vi "subDAQ_SetFilterSet.vi"(6 "Ti-E cluster":T3, 7 "Filterset cluster":T1={"filter set (row)"=18, "Light control ref"=refnum, "Confocal Refnum"=refnum, "DAQ ports"={"Lasers DO lines"=["Dev2/port0/line0", "Dev2/port0/line1", "Dev2/port0/line2", "Dev2/port0/line3", "Dev2/port0/line4", "Dev2/port0/line5"], "Lasers AO lines"=["Dev2/ao0", "Dev2/ao1", "Dev2/ao2", "Dev2/ao3", "Dev2/ao4", "Dev2/ao5"], "Patch AO line"="Dev1/ao1", "Patch AI lines 1"={"Patch scaled output"="Dev1/ai13", "Patch 10 V_m "="Dev1/ai8"}, "Camera timing DI"="Dev1/port0/line23", "Dev1 timing DO "="Dev1/port0/line18", "Dev1 trigger source"="/Dev1/PFI0", "Dev2 trigger source"="/Dev2/PFI0", "LED line"="Dev1/port0/line8", "Global Shutter line"="Dev1/port0/line9", "Patch AI lines 2"={"Cell capacitance"="Dev1/ai9", "Mode"="Dev1/ai10", "Frequency"="Dev1/ai11", "Gain"="Dev1/ai12"}}, "Confocal VISA Setting"="COM1"}, 8 "error in":errorcluster) -> (0 "error out":errorcluster)   [LabVIEW 2015]
uses:
  <vilib>/Analysis/Matrix/Datatypes/RealMatrix.ctl
  <vilib>/Analysis/Matrix/NI_Matrix.lvlib
panel:
  out "Light control":T2={"Filter Set"=17, "Lasers DO"=[TRUE, FALSE, FALSE, FALSE, FALSE, FALSE], "Lasers AO (V)"=[0.3, 0.3, 0.3, 0.3, 0.3, 0.3], "LED"=FALSE, "Global"=TRUE} {"Lasers AO (V)" min=0.0 max=5.0 step=0.01 scale=0.0..5.0 scale format="%#1.2f"; "Filter Set" items=["R-QuasAr", "R-Cy5", "R-mCherry", "R-mOrange", "R-GFP", "R-CFP/DAPI", "R-BFP", "R-LED", "SDC-Cy5", "SDC-mCherry", "SDC-mO2", "SDC-GFP", "SDC-CFP/DAPI", "SDC-BFP", "SDC-LED"]}
  in  "Filter Set Table":T4=[[0.0, 5.0, 2.0, 6.0, 6.0, 1.0, 0.0], [1.0, 0.0, 2.0, 6.0, 6.0, 1.0, 0.0], [2.0, 1.0, 2.0, 2.0, 6.0, 1.0, 0.0], [3.0, 2.0, 1.0, 3.0, 6.0, 1.0, 0.0], [4.0, 3.0, 2.0, 1.0, 6.0, 1.0, 0.0], [5.0, 4.0, 2.0, 5.0, 6.0, 1.0, 0.0], [6.0, 4.0, 2.0, 5.0, 6.0, 1.0, 0.0], [7.0, -1.0, 6.0, 4.0, 6.0, 0.0, 1.0], [8.0, 0.0, 3.0, 4.0, 4.0, 0.0, 0.0], [9.0, 1.0, 3.0, 4.0, 3.0, 0.0, 0.0], [10.0, 2.0, 3.0, 4.0, 5.0, 0.0, 0.0], [11.0, 3.0, 3.0, 4.0, 2.0, 0.0, 0.0], [12.0, 4.0, 3.0, 4.0, 1.0, 0.0, 0.0], [13.0, 4.0, 3.0, 4.0, 1.0, 0.0, 0.0], [14.0, -1.0, 6.0, 4.0, 6.0, 0.0, 1.0], [15.0, 3.0, 3.0, 4.0, 3.0, 0.0, 0.0], [16.0, 3.0, 2.0, 2.0, 6.0, 1.0, 0.0], [17.0, -1.0, 2.0, 4.0, 6.0, 1.0, 0.0], [18.0, -1.0, 1.0, 3.0, 6.0, 0.0, 0.0]]
  # "Change Filter set according to the Table"
  # "Filter Set Table"
  # "No.    Laser  Top   Btm    FW    Glb    LED"
  # "Red"
  # "637"
  # "561"
  # "488"
  # "405"
  # "532"
  # "637"
  # "561"
  # "532"
  # "488"
  # "405"
  # "Red"
  # "Red"
  # "637"
  # "561"
  # "488"
  # "405"
  # "532"
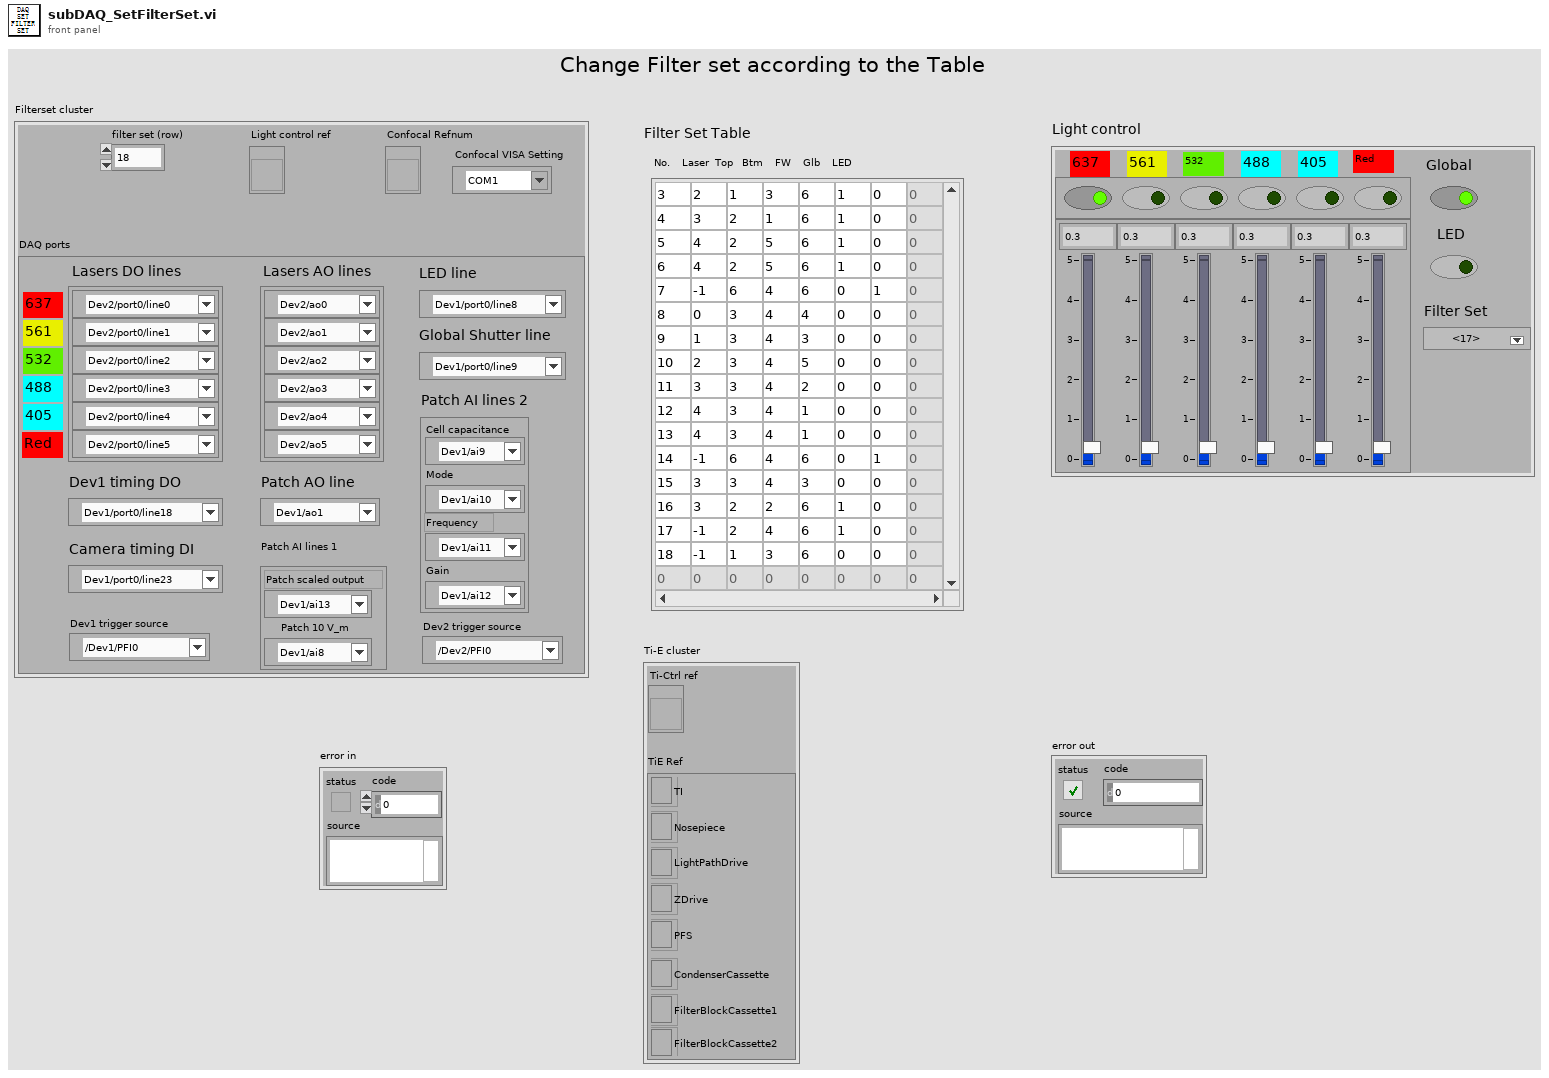
[diagram p1: front panel]
types:
  T1 = cluster{"filter set (row)":i32, "Light control ref":refnum<vi>, "Confocal Refnum":refnum<vi>, "DAQ ports":cluster{"Lasers DO lines":tag[], "Lasers AO lines":tag[], "Patch AO line":tag, "Patch AI lines 1":cluster{"Patch scaled output":tag, "Patch 10 V_m ":tag}, "Camera timing DI":tag, "Dev1 timing DO ":tag, "Dev1 trigger source":tag, "Dev2 trigger source":tag, "LED line":tag, "Global Shutter line":tag, "Patch AI lines 2":cluster{"Cell capacitance":tag, "Mode":tag, "Frequency":tag, "Gain":tag}}, "Confocal VISA Setting":refnum<visa-resource-name>}
  T2 = cluster{"Filter Set":i32, "Lasers DO":bool[], "Lasers AO (V)":dbl[], "LED":bool, "Global":bool}
  T3 = cluster{"Ti-Ctrl ref":refnum<vi>, "TiE Ref":cluster{"TI":refnum<k7>, "Nosepiece":refnum<k7>, "LightPathDrive":refnum<k7>, "ZDrive":refnum<k7>, "PFS":refnum<k7>, "CondenserCassette":refnum<k7>, "FilterBlockCassette1":refnum<k7>, "FilterBlockCassette2":refnum<k7>}}
  T4 = typedef "NI_Matrix.lvlib/RealMatrix.ctl" = dbl[][]
  T5 = cluster{"SDC shutter":bool, "Filter wheel":u16, "FW speed":i32, "Disk spinning":bool, "Disk speed (rpm)":dbl}
  T6 = cluster{"Obj":u16, "Cube Bottom":u16, "Cube Top":u16, "PFS-Ctrl":cluster{"PFS IO":bool, "PSF Err":bool, "PSF Pos":u32}, "Z-Ctrl":cluster{"Z-pos":dbl, "Home":bool, "Sensitivity":u8}, "Condenser":u16, "Lightpath":enum32{"EYE", "L100", "R100", "L80"}}
  T7 = cluster{"TI":refnum<k7>, "Nosepiece":refnum<k7>, "LightPathDrive":refnum<k7>, "ZDrive":refnum<k7>, "PFS":refnum<k7>, "CondenserCassette":refnum<k7>, "FilterBlockCassette1":refnum<k7>, "FilterBlockCassette2":refnum<k7>}
  T8 = cluster{"Lasers DO lines":tag[], "Lasers AO lines":tag[], "Patch AO line":tag, "Patch AI lines 1":cluster{"Patch scaled output":tag, "Patch 10 V_m ":tag}, "Camera timing DI":tag, "Dev1 timing DO ":tag, "Dev1 trigger source":tag, "Dev2 trigger source":tag, "LED line":tag, "Global Shutter line":tag, "Patch AI lines 2":cluster{"Cell capacitance":tag, "Mode":tag, "Frequency":tag, "Gain":tag}}
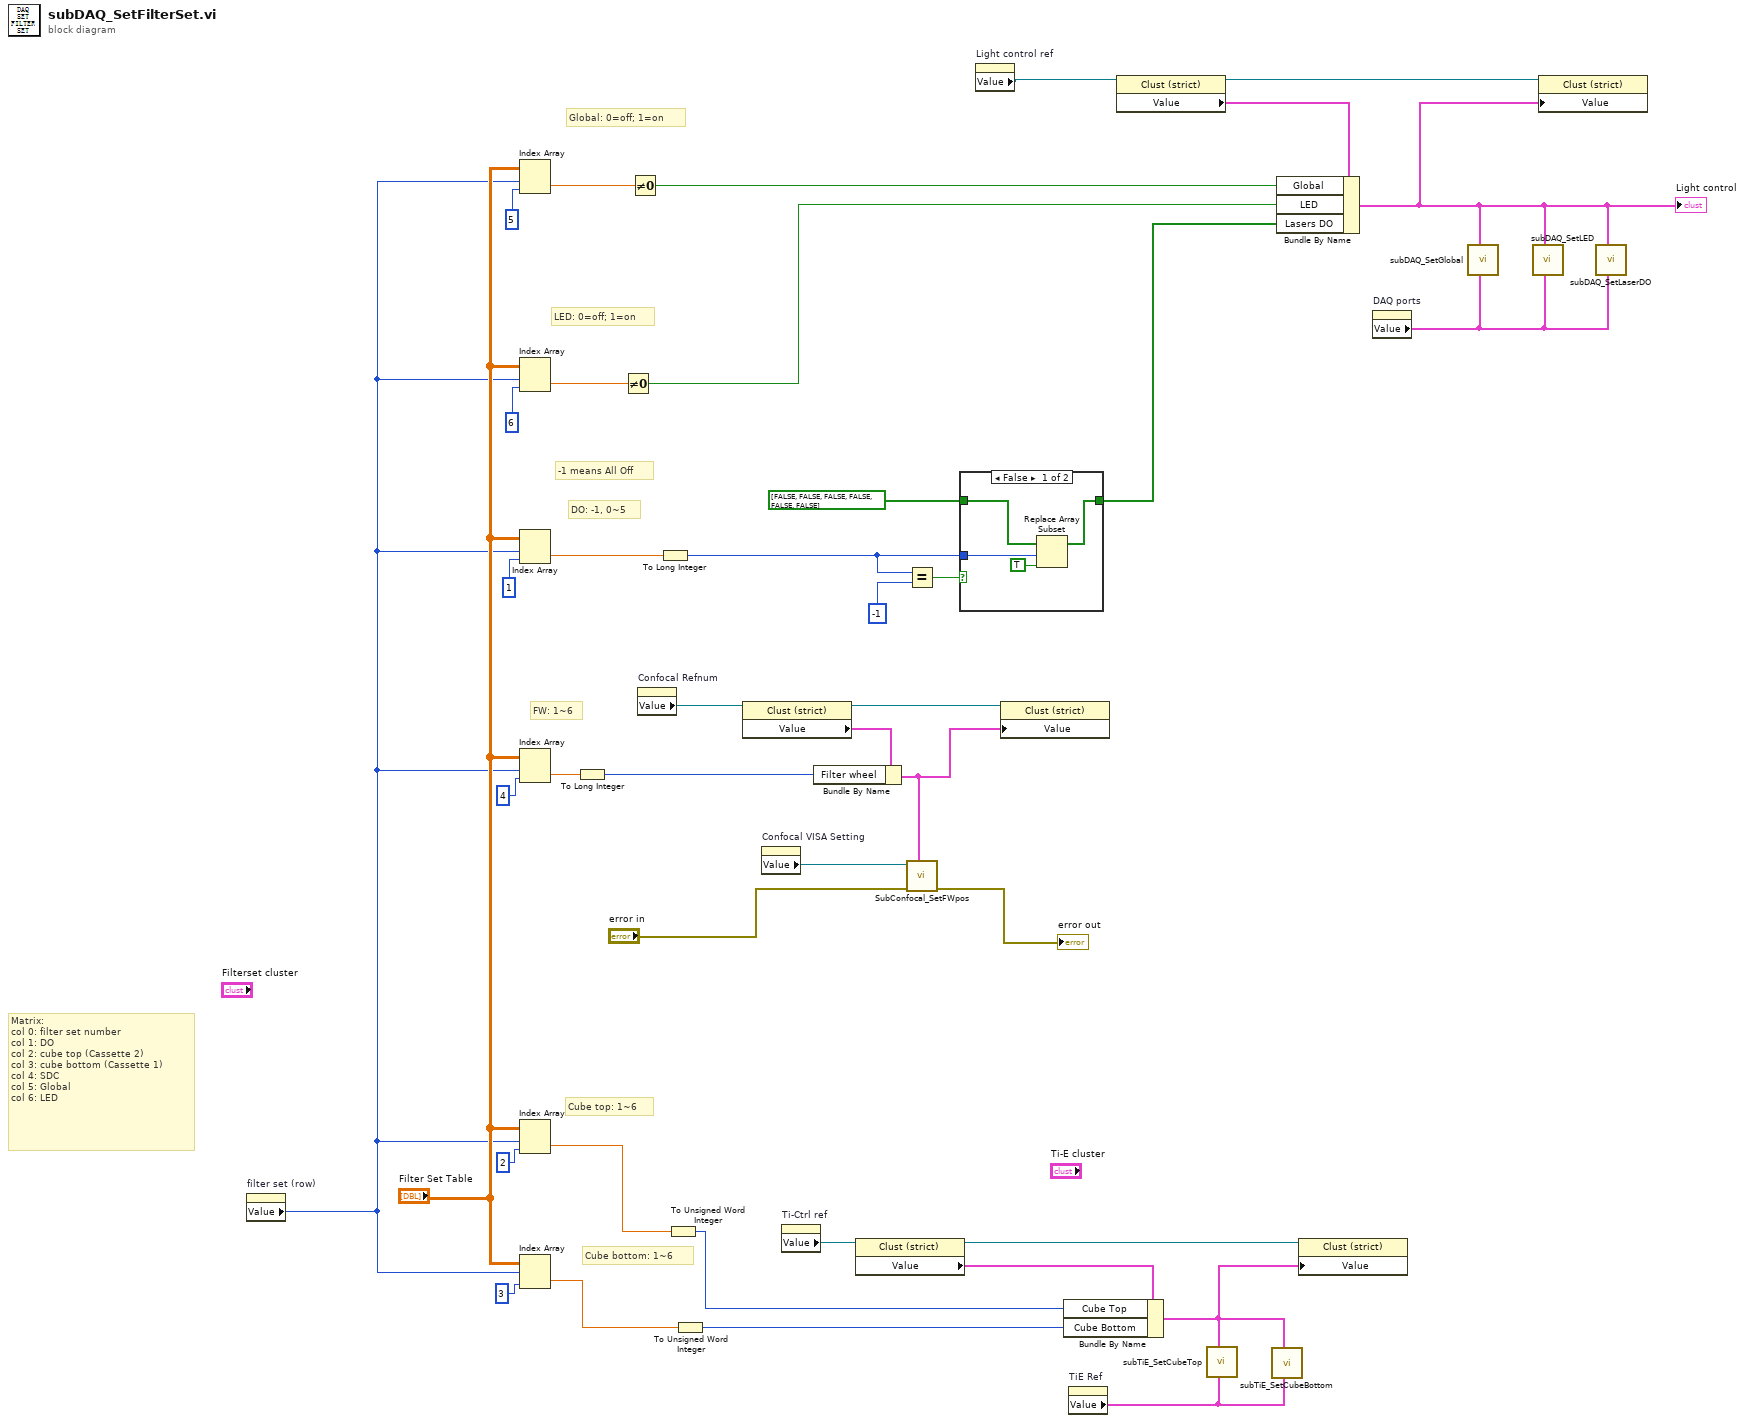
[diagram p0: block diagram]
diagram:
  # "-1 means All Off"
  # "LED: 0=off; 1=on"
  # "Global: 0=off; 1=on"
  # "FW: 1~6"
  # "Cube bottom: 1~6"
  # "Cube top: 1~6"
  # "DO: -1, 0~5"
  # "Matrix:\ncol 0: filter set number\ncol 1: DO\ncol 2: cube top (Cassette 2)\ncol 3: cube bottom (Cassette 1)\ncol 4: SDC\ncol 5: Global\ncol 6: LED"
  n1 = property on="filter set (row)" class="DigNum (strict)"() -> ("Value"=w1:i32)  [unwired: 2 in, 2 out]
  n2 = Index Array(array="Filter Set Table", index (row)=w1, index (col)=5) -> (element=w23:dbl)
  n3 = Index Array(array="Filter Set Table", index (row)=w1, index (col)=6) -> (element=w20:dbl)
  n4 = Index Array(array="Filter Set Table", index (row)=w1, index (col)=1) -> (element=w38:dbl)
  n5 = Index Array(array="Filter Set Table", index (row)=w1, index (col)=4) -> (element=w27:dbl)
  n6 = Index Array(array="Filter Set Table", index (row)=w1, index (col)=2) -> (element=w30:dbl)
  n7 = Index Array(array="Filter Set Table", index (row)=w1, index (col)=3) -> (element=w29:dbl)
  n8 = To Long Integer(number=w27) -> (32bit integer=w10:i32)
  n9 = Not Equal To 0?(x=w20) -> (x != 0?=w15:bool)
  n10 = Not Equal To 0?(x=w23) -> (x != 0?=w16:bool)
  n11 = property on="Confocal Refnum" class="LVObjRef (strict)"() -> ("Value"=w3:refnum<vi>)  [unwired: 2 in, 2 out]
  n12 = To Long Integer(number=w38) -> (32bit integer=w24:i32)
  n13 = To Unsigned Word Integer(number=w30) -> (unsigned 16bit integer=w33:u16)
  n14 = To Unsigned Word Integer(number=w29) -> (unsigned 16bit integer=w32:u16)
  n15 = property class="Clust (strict)"(reference=w3) -> (reference out=w9:refnum<vi>, "Value"=w11:T5)  [unwired: 1 in, 1 out]
  n16 = property on="Confocal VISA Setting" class="VISAName"() -> ("Value"=w2:refnum<visa-resource-name>)  [unwired: 2 in, 2 out]
  n17 = property on="Ti-Ctrl ref" class="LVObjRef (strict)"() -> ("Value"=w6:refnum<vi>)  [unwired: 2 in, 2 out]
  n18 = Bundle By Name(cluster=w11, "Filter wheel"=w10) -> (w8:T5)
  n19 = property class="Clust (strict)"(reference=w6) -> (reference out=w31:refnum<vi>, "Value"=w34:T6)  [unwired: 1 in, 1 out]
  n20 = Equal?(x=w24, y=-1) -> (x = y?=w26:bool)
  n21 = call "SubConfocal_SetFWpos.vi"("Confocal scanner"=w8, "Error In"="error in", "Confocal line (VISA IN)"=w2) -> ("Error out"=→"error out":errorcluster)  [unwired: 7 in, 1 out]
  n22 = case shown="False" w26 {
    tunnel: bool[] [FALSE, FALSE, FALSE, FALSE, FALSE, FALSE] ("initialized array") -> [w45 w46]
    tunnel: [w43 w46] -> w12
    tunnel: w24 -> [w42 _]
    frame False {
      n23 = Replace Array Subset(array=w45, new element=TRUE ("new element/subarray"), index=w42) -> (w43:bool[])
    }
    frame True {
      # "All OFF"
    }
  }
  n24 = property on="Light control ref" class="LVObjRef (strict)"() -> ("Value"=w5:refnum<vi>)  [unwired: 2 in, 2 out]
  n25 = property class="Clust (strict)"(reference=w9, "Value"=w8) -> ()  [unwired: 1 in, 2 out]
  n26 = Bundle By Name(cluster=w34, "Cube Top"=w33, "Cube Bottom"=w32) -> (w19:T6)
  n27 = property on="TiE Ref" class="Clust (strict)"() -> ("Value"=w7:T7)  [unwired: 2 in, 2 out]
  n28 = property class="Clust (strict)"(reference=w5) -> (reference out=w18:refnum<vi>, "Value"=w17:T2)  [unwired: 1 in, 1 out]
  n29 = call "subTiE_SetCubeTop.vi"("Ref"=w7, "TI-Ctrl"=w19) -> ()  [unwired: 10 in]
  n30 = call "subTiE_SetCubeBottom.vi"("Ref"=w7, "TI-Ctrl"=w19) -> ()  [unwired: 10 in]
  n31 = Bundle By Name(cluster=w17, "Global"=w16, "LED"=w15, "Lasers DO"=w12) -> (w14:T2)
  "Light control" <- w14
  n32 = property class="Clust (strict)"(reference=w31, "Value"=w19) -> ()  [unwired: 1 in, 2 out]
  n33 = property on="DAQ ports" class="Clust (strict)"() -> ("Value"=w4:T8)  [unwired: 2 in, 2 out]
  n34 = call "subDAQ_SetGlobal.vi"("DAQ ports"=w4, "Light control (All off)"=w14) -> ()  [unwired: 9 in, 1 out]
  n35 = call "subDAQ_SetLED.vi"("DAQ ports"=w4, "Light control (All Off)"=w14) -> ()  [unwired: 9 in, 1 out]
  n36 = property class="Clust (strict)"(reference=w18, "Value"=w14) -> ()  [unwired: 1 in, 2 out]
  n37 = call "subDAQ_SetLaserDO.vi"("DAQ ports"=w4, "Light control (All off)"=w14) -> ()  [unwired: 9 in, 1 out]
